vi "Read Product Selected Ref.vi"(11 "Products Picker in":refnum<class "Products Picker.lvclass">) -> (2 "Product Selected Ref":refnum<vi>, 3 "Products Picker out":refnum<class "Products Picker.lvclass">)   [LabVIEW 2020, in "Products Picker.lvlib" / "Products Picker.lvclass"]
uses:
  Products Picker.lvclass
  Products Picker.lvclass/Products Picker.ctl
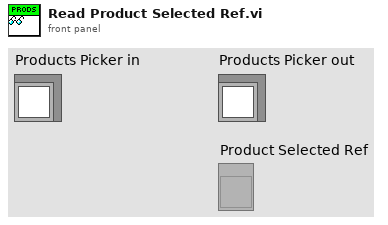
[diagram p1: front panel]
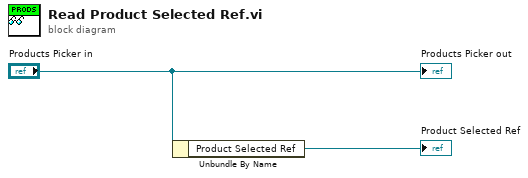
[diagram p0: block diagram]
diagram:
  n1 = Unbundle By Name("Products Picker in") -> ("Product Selected Ref"=→"Product Selected Ref":refnum<vi>)
  "Products Picker out" <- "Products Picker in"
